vi "Create Plugin.vi"(5 "Debug Flags":refnum<class "Debug Flags.lvclass">, 7 "transceiver count":i32, 8 "error in (no error)":errorcluster, 9 "component classes":refnum<class>[](array[class]), 10 "Plugin Configuration":T1={"name"="", "class"="", "cycle timing"={"priority"=0, "decimation"=1, "offset"=0}, "Transfer Groups"=[], "settings"=[]}, 11 "Transfer Groups":refnum<class "Transfer Group.lvclass">[](array[class])) -> (0 "error out":errorcluster, 2 "Transceiver":refnum<class "Transceiver.lvclass">, 3 "Plugin out":refnum<class "Plugin.lvclass">)   [LabVIEW 2017, in "DSF Core.lvlib" / "Plugin.lvclass"]
uses:
  Plugin.lvclass
  Transfer Group/Transfer Group.lvclass
  Debug/Debug Flags/Debug Flags.lvclass
  DSF Configuration API/Public/Controls/DSF Engine Plugin Configuration.ctl
  DSF Configuration API/Public/Controls/DSF Timing Info.ctl
  DSF Configuration API/Public/Controls/DSF Engine Transfer Group Configuration.ctl
  DSF Configuration API/Public/Controls/DSF Direction.ctl
  DSF Configuration API/Public/Controls/DSF Engine Transfer Configuration.ctl
  DSF Configuration API/Public/Controls/DSF Byte Order.ctl
  DSF Configuration API/Public/Controls/DSF Engine Channel Configuration.ctl
  DSF Configuration API/Public/Controls/DSF Data Type.ctl
  DSF Configuration API/Public/Controls/DSF Settings Info.ctl
  Transceiver/Transceiver.lvclass
  Plugin.lvclass/Plugin.ctl
  Timing/Timing.lvclass
  DSF Core.lvlib
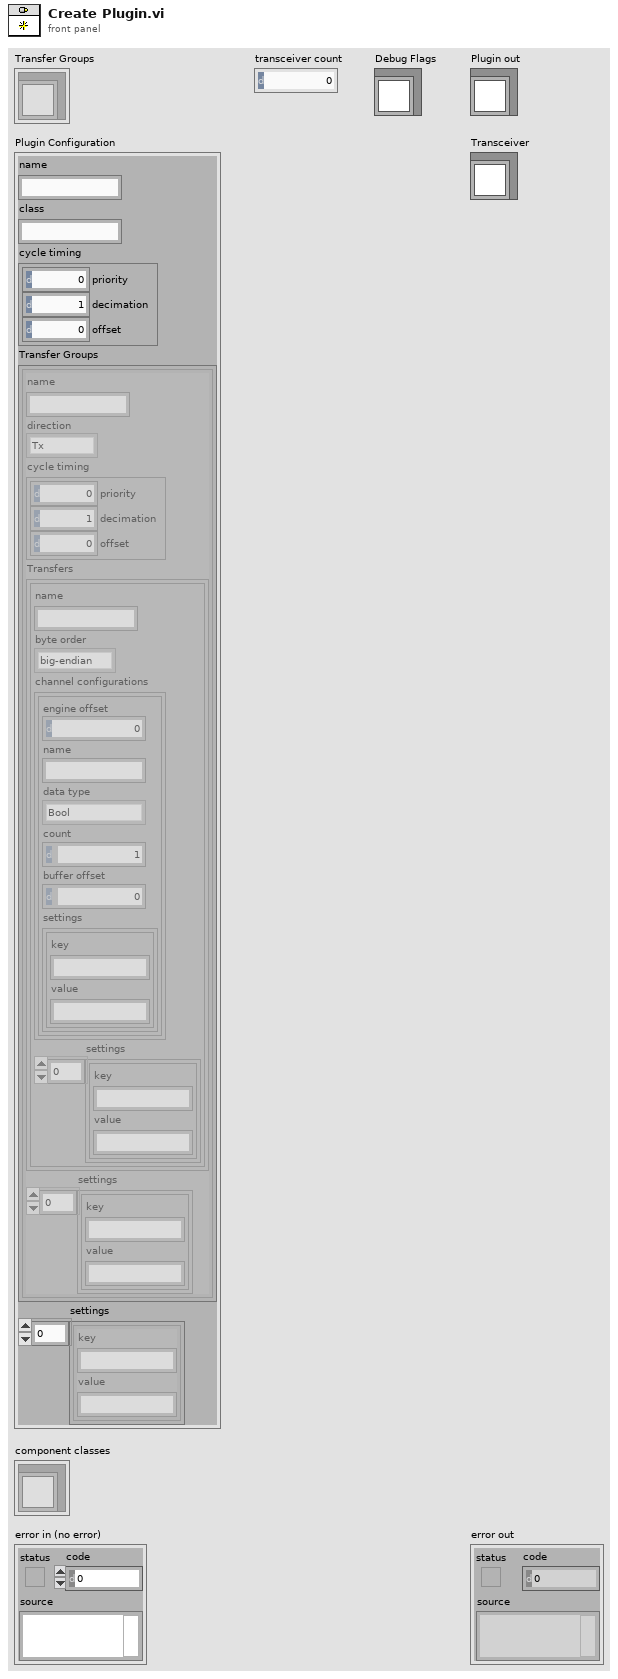
[diagram p1: front panel]
types:
  T1 = typedef "DSF Core.lvlib/DSF Engine Plugin Configuration.ctl" = cluster{"name":string, "class":string, "cycle timing":T2, "Transfer Groups":T3[], "settings":T9}
  T2 = typedef "DSF Core.lvlib/DSF Timing Info.ctl" = cluster{"priority":u64, "decimation":u64, "offset":u64}
  T3 = typedef "DSF Core.lvlib/DSF Engine Transfer Group Configuration.ctl" = cluster{"name":string, "direction":T4, "cycle timing":T2, "Transfers":T5[], "settings":T9}
  T4 = typedef "DSF Core.lvlib/DSF Direction.ctl" = enum8{"Tx", "Rx"}
  T5 = typedef "DSF Core.lvlib/DSF Engine Transfer Configuration.ctl" = cluster{"name":string, "byte order":T6, "channel configurations":T7[], "settings":T9}
  T6 = typedef "DSF Core.lvlib/DSF Byte Order.ctl" = enum8{"big-endian", "little-endian"}
  T7 = typedef "DSF Core.lvlib/DSF Engine Channel Configuration.ctl" = cluster{"engine offset":u64, "name":string, "data type":T8, "count":u64, "buffer offset":u64, "settings":T9}
  T8 = typedef "DSF Core.lvlib/DSF Data Type.ctl" = enum8{"Bool", "SGL", "DBL", "I8", "I16", "I32", "I64", "U8", "U16", "U32", "U64"}
  T9 = typedef "DSF Core.lvlib/DSF Settings Info.ctl" = cluster{"key":string, "value":string}[]
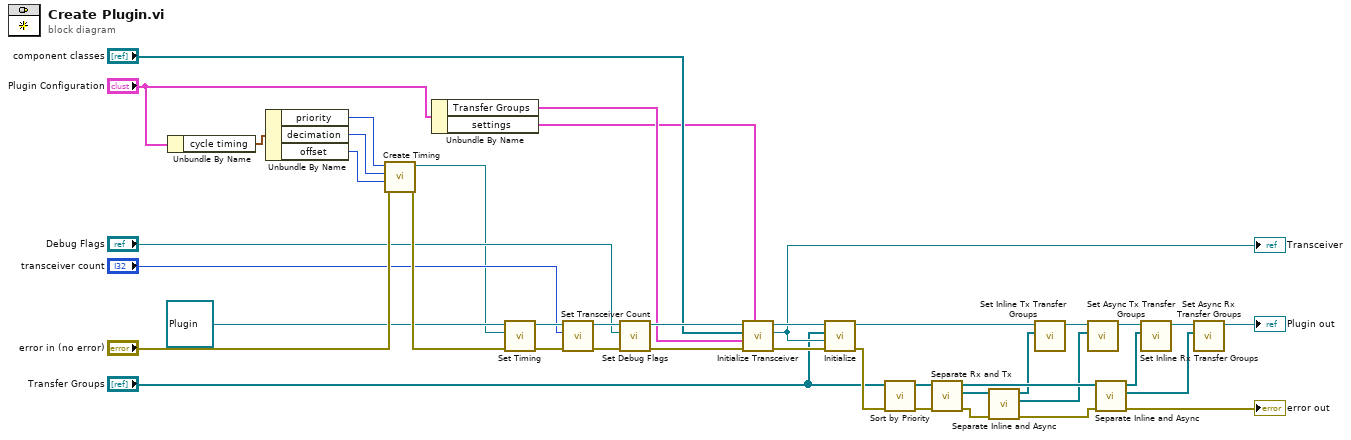
[diagram p0: block diagram]
diagram:
  n1 = Unbundle By Name("Plugin Configuration") -> ("cycle timing"=w1:T2)
  n2 = Unbundle By Name(w1) -> ("priority"=w12:u64, "decimation"=w13:u64, "offset"=w14:u64)
  n3 = call "Create Timing.vi"("error in (no error)"="error in (no error)", "Offset"=w14, "Decimation"=w13, "Priority"=w12) -> ("error out"=w37:errorcluster, "Timing"=w11:refnum<class "Timing.lvclass">)  [unwired: 6 in]
  n4 = Unbundle By Name("Plugin Configuration") -> ("Transfer Groups"=w4:T3[], "settings"=w3:T9)
  n5 = call "Set Timing.vi"("Timing"=w11, "Plugin in"=refnum<class "Plugin.lvclass"> refnum) -> ("Plugin out"=w34:refnum<class "Plugin.lvclass">)  [unwired: 9 in]
  n6 = call "Set Transceiver Count.vi"("transceiver count"="transceiver count", "Plugin in"=w34) -> ("Plugin out"=w21:refnum<class "Plugin.lvclass">)  [unwired: 9 in]
  n7 = call "Set Debug Flags.vi"("Debug Flags"="Debug Flags", "Plugin in"=w21) -> ("Plugin out"=w10:refnum<class "Plugin.lvclass">)  [unwired: 9 in]
  n8 = call "Initialize Transceiver.vi"("transceiver settings"=w3, "error in (no error)"=w37, "Transfer Groups Configurations"=w4, "component classes"="component classes", "Plugin in"=w10) -> ("error out"=w6:errorcluster, "Transceiver"=w7:refnum<class "Transceiver.lvclass">, "Plugin out"=w9:refnum<class "Plugin.lvclass">)  [unwired: 4 in]
  "Transceiver" <- w7
  n9 = call "Initialize.vi"("error in (no error)"=w6, "Transceiver"=w7, "Transfer Groups"="Transfer Groups", "Plugin in"=w9) -> ("error out"=w17:errorcluster, "Plugin out"=w19:refnum<class "Plugin.lvclass">)  [unwired: 6 in]
  n10 = call "Sort by Priority.vi"("error in (no error)"=w17, "Transfer Groups"="Transfer Groups") -> ("error out"=w36:errorcluster, "sorted Transfer Groups"=w35:refnum<class "Transfer Group.lvclass">[])  [unwired: 8 in]
  n11 = call "Separate Rx and Tx.vi"("error in (no error)"=w36, "Transfer Groups"=w35) -> ("error out"=w32:errorcluster, "Tx Transfer Groups"=w31:refnum<class "Transfer Group.lvclass">[], "Rx Transfer Groups"=w30:refnum<class "Transfer Group.lvclass">[])  [unwired: 7 in]
  n12 = call "Separate Inline and Async.vi"("error in (no error)"=w32, "Transfer Groups"=w31) -> ("error out"=w29:errorcluster, "Async Transfer Groups"=w27:refnum<class "Transfer Group.lvclass">[], "Inline Transfer Groups"=w28:refnum<class "Transfer Group.lvclass">[])  [unwired: 7 in]
  n13 = call "Set Inline Tx Transfer Groups.vi"("Inline Tx Transfer Groups"=w28, "Plugin in"=w19) -> ("Plugin out"=w26:refnum<class "Plugin.lvclass">)  [unwired: 9 in]
  n14 = call "Set Async Tx Transfer Groups.vi"("Async Tx Transfer Groups"=w27, "Plugin in"=w26) -> ("Plugin out"=w24:refnum<class "Plugin.lvclass">)  [unwired: 9 in]
  n15 = call "Separate Inline and Async.vi"("error in (no error)"=w29, "Transfer Groups"=w30) -> ("error out"=→"error out":errorcluster, "Async Transfer Groups"=w22:refnum<class "Transfer Group.lvclass">[], "Inline Transfer Groups"=w25:refnum<class "Transfer Group.lvclass">[])  [unwired: 7 in]
  n16 = call "Set Inline Rx Transfer Groups.vi"("Inline Rx Transfer Groups"=w25, "Plugin in"=w24) -> ("Plugin out"=w23:refnum<class "Plugin.lvclass">)  [unwired: 9 in]
  n17 = call "Set Async Rx Transfer Groups.vi"("Async Rx Transfer Groups"=w22, "Plugin in"=w23) -> ("Plugin out"=→"Plugin out":refnum<class "Plugin.lvclass">)  [unwired: 9 in]
